vi "ProcessCommand.vi"(5 "Ctl Refnum":refnum<vi>, 7 "Command":variant, 8 "error in (no error)":errorcluster, 9 "Data":T1=variant(string "Default"), 10 "Queue with Cluster Reference":T2, 11 "EVM Command in":refnum<class "EVMQueueCommand.lvclass">) -> (0 "error out":errorcluster, 2 "Queue (dup)":T2, 3 "EVM Command out":refnum<class "EVMQueueCommand.lvclass">)   [LabVIEW 2010, in "EVMQueueCommand.lvclass"]
doc: "This VI serves as the dynamic dispatch VI for queueing the correct command for processing.\n\nInputs:\nEVMQueueCommand object - object determines which enqueueing function is called. Valid objects are:\n - EVMQueueCommand object - object used for NO OP cases (do no enqueue anything)\n - Shell Command object - object used for commands from the shell\n - UserInput Command object - object used for commands from the user interface\n - Internal State Command object - object used for commands within the plugin action loop\n\nCommand - variant data type. Not required input for all objects\n - EVMQueueCommand object - not required\n - Shell Command object - SignalCommandControl typedef\n - UserInput Command object - valid as string (for Not A Ref on control reference input)\n - Internal State Command object - valid as string (for Not A Ref on control reference input)\n\nData - variant (not valid for general case); used to input data to the queue with the command (this overrides the control current value normally placed in the queue)\n\nQueue with Cluster Reference - reference to the EVM queue for inserting commands\n\nCtl Refnum -\n(valid for UserInput Command and Internal State Command objects) \n - UserInput Command - reference to the control that triggered the event; Not A Ref constant allows user defined string constants to be wired to Data input\n - Internal State Command - Not A Ref constant allows user defined string constants to be wired to Data input\nerror in - error input cluster\n\nOutputs:\nEVM Command out - input object passed through\nQueue (dup) - input queue reference passed through\nerror out - error output cluster"
uses:
  EVMQueueCommand.lvclass
  <userlib>/Common/Queue with Cluster/TYP_Queue with Cluster Reference.ctl
  Controls/TYP_VariantDefault.ctl
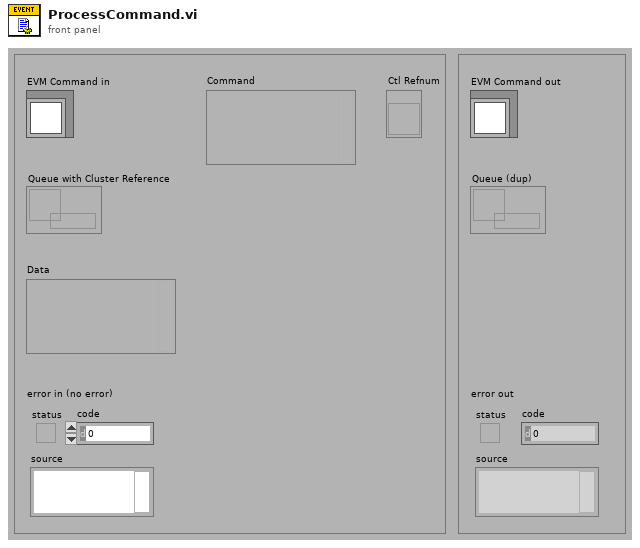
[diagram p1: front panel]
types:
  T1 = typedef "TYP_VariantDefault.ctl" = variant
  T2 = typedef "TYP_Queue with Cluster Reference.ctl" = refnum<queue>
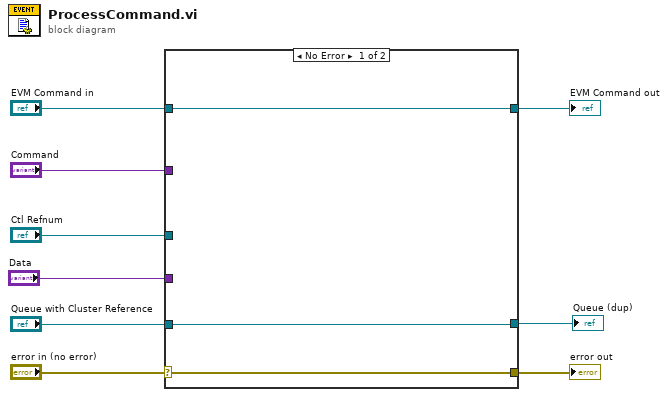
[diagram p0: block diagram]
diagram:
  n1 = case shown="No Error" "error in (no error)" {
    selector: "error in (no error)" -> [w11 w15]
    tunnel: [w11 w15] -> w8
    tunnel: [w12 w14] -> w6
    tunnel: "EVM Command in" -> [w12 w14]
    tunnel: [w10 w13] -> w4
    tunnel: "Queue with Cluster Reference" -> [w10 w13]
    tunnel: "Command" -> [_ _]
    tunnel: "Ctl Refnum" -> [_ _]
    tunnel: "Data" -> [_ _]
    frame No Error {
    }
    frame Error {
    }
  }
  "error out" <- w8
  "EVM Command out" <- w6
  "Queue (dup)" <- w4
